vi "Peer to Peer - Basic.vi"() -> ()   [LabVIEW 2023]
uses:
  <vilib>/userDefined/High Color/nirio_resource_hc.ctl
  <vilib>/userDefined/niP2PState.ctl
  <vilib>/FPGAPlugInAG/PXIe-7965R/niLvFpga_Open_PXIe-7965R.vi
  <vilib>/FPGAPlugInAG/PXIe-7965R/niLvFpga_P2PGetEndpoint_PXIe-7965R.vi
  <vilib>/Utility/error.llb/Error Cluster From Error Code.vi
  <vilib>/rvi/errors/niLvFpgaAdjustHostInterfaceError.vi
  <vilib>/FPGAPlugInAG/PXIe-7965R/niLvFpga_Close_PXIe-7965R.vi
  <vilib>/rvi/interface/nirviOpenFPGA/nirviOpenFPGA.xnode
  FPGA Bitfiles/PeerToPeerW_PXIe-7965R.lvbitx
  FPGA Bitfiles/PeerToPeerR_PXIe-7965R.lvbitx
  <vilib>/rvi/interface/nirviMethod/nirviMethod.xnode
  <vilib>/rvi/interface/nirviReadWriteControl/nirviReadWriteControl.xnode
  <vilib>/rvi/interface/nirviCloseFPGA/nirviCloseFPGA.xnode
  <resource>/objmgr/PeerToPeerStream.rc
  <vilib>/rvi/errors/niLvFpgaMergeErrorWithErrorCode.vi
  NiFpgaLv.dll
panel:
  out "Stream State":T1
  in  "Reader":T2="RIO1"
  in  "Writer":T2="RIO0"
  out "Transfer Rate (MB/s)":dbl format="%.3f"
  out "Data Valid?":bool
  out "DataRead":u64
  out "Data Expected":u64
  in  "stop":bool
  in  "Enable":bool
  in  "Flush And Disable":bool
  # "This example shows how to setup and configure a peer to \npeer stream between two PXIe FlexRIO boards. There is a \npeer to peer stream created between the writer and reader \ndevice and once it is enabled, the writer will write a counter \nvalue to the reader. The reader will validate the received\ndata against it's own counter to ensure they match. In \naddition, this example measures throughput of the stream."
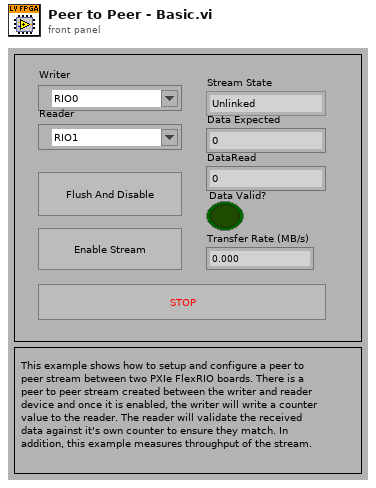
[diagram p1: front panel]
types:
  T1 = typedef "niP2PState.ctl" = enum32{"Unlinked", "Disabled", "Enabled", "Flushing"}
  T2 = typedef "nirio_resource_hc.ctl" = tag
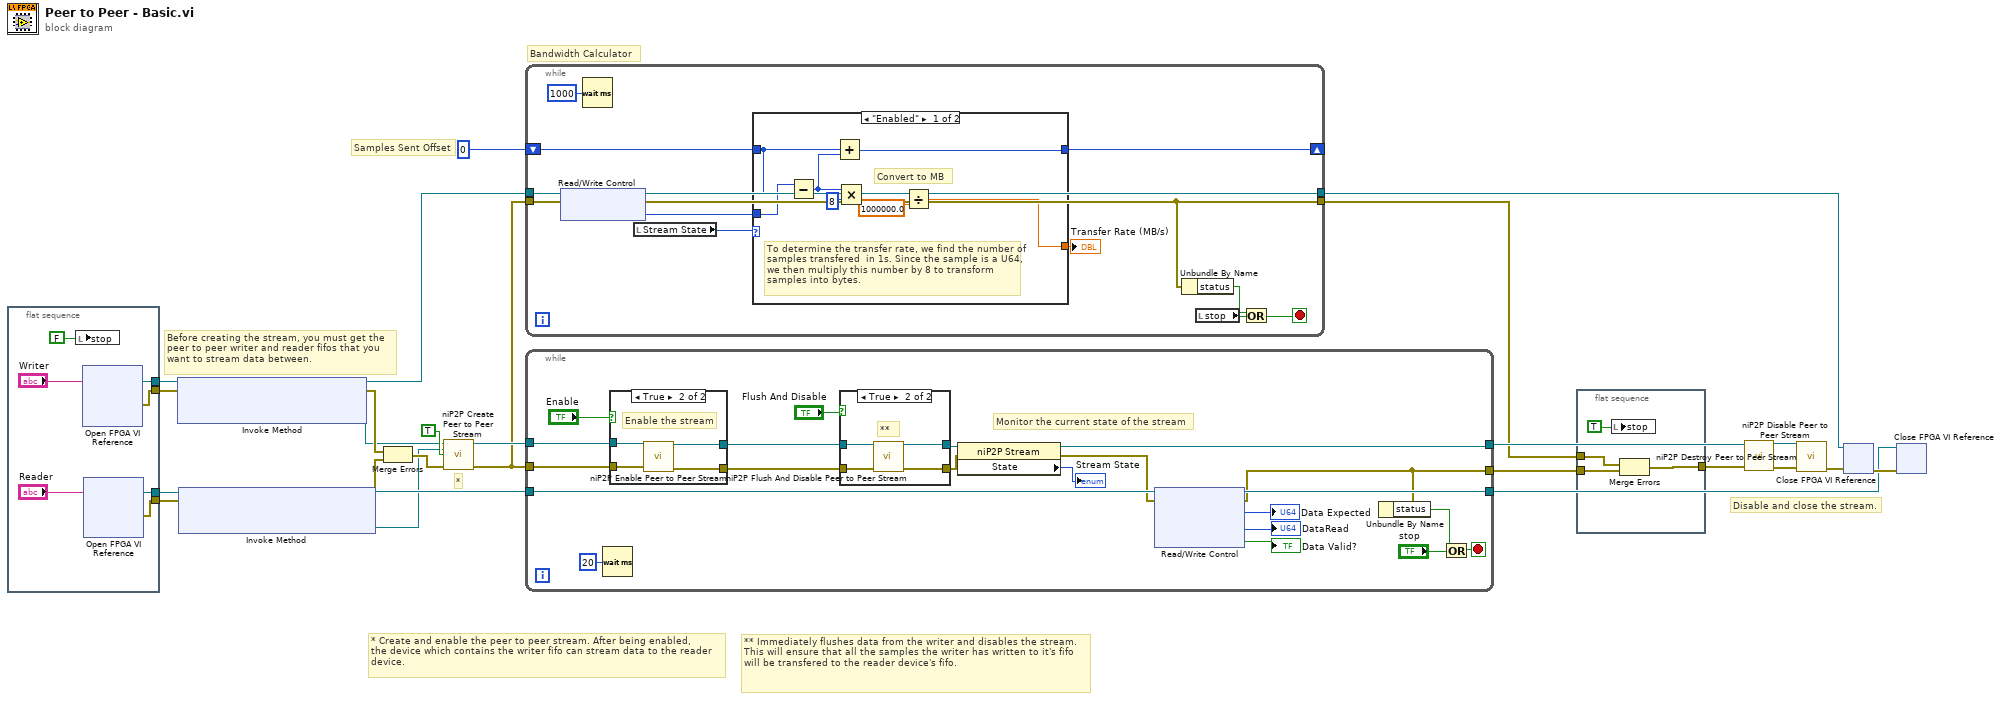
[diagram p0: block diagram]
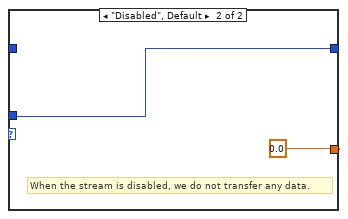
[diagram p2: hidden frame]
diagram:
  # "Bandwidth Calculator"
  # "Samples Sent Offset"
  # "** Immediately flushes data from the writer and disables the stream. \nThis will ensure that all the samples the writer has written to it's fifo \nwill be transfered to the reader device's fifo."
  # "Disable and close the stream."
  # "*"
  # "* Create and enable the peer to peer stream. After being enabled, \nthe device which contains the writer fifo can stream data to the reader\ndevice."
  # "Before creating the stream, you must get the \npeer to peer writer and reader fifos that you \nwant to stream data between."
  n1 = flat-sequence {
    tunnel: [w32] -> w6
    tunnel: [w31] -> w5
    tunnel: [w30] -> w25
    tunnel: [w29] -> w24
    frame #0 {
      n2 = local write "stop"(FALSE ("stop")) -> ()
      n3 = xnode "Open FPGA VI Reference"("resource name"="Writer") -> ("FPGA VI Reference Out"=w32:refnum<k20>, "error out"=w31:errorcluster)  [unwired: 1 in]
      n4 = xnode "Open FPGA VI Reference"("resource name"="Reader") -> ("FPGA VI Reference Out"=w30:refnum<k20>, "error out"=w29:errorcluster)  [unwired: 1 in]
    }
  }
  n5 = xnode "Invoke Method"("FPGA VI Reference In"=w6, "error in"=w5) -> ("FPGA VI Reference Out"=w4:refnum<k20>, "error out"=w3:errorcluster, "Writer"=w2:refnum<k20>)
  n6 = xnode "Invoke Method"("FPGA VI Reference In"=w25, "error in"=w24) -> ("FPGA VI Reference Out"=w23:refnum<k20>, "error out"=w22:errorcluster, "Reader"=w1:refnum<k20>)
  n7 = Merge Errors(w3, w22) -> (w21:errorcluster)
  n8 = call <vilib>:"niP2P Create Peer to Peer Stream.vi"("writer"=w2, "reader"=w1, "enable stream (T)"=TRUE, "error in (no error)"=w21) -> ("stream session"=w13:refnum<k20>, "error out"=w12:errorcluster)  [unwired: 10 in]
  n9 = while {
    tunnel: w4 -> [w39]
    tunnel: w12 -> [w38]
    shift-right: [w40] -> _
    shift-left: u64 0 -> [w41]
    tunnel: [w35] -> w8
    tunnel: [w37] -> w7
    stop <- w43 stop-if-true
    n10 = xnode "Read/Write Control"("FPGA VI Reference In"=w39, "error in"=w38) -> ("FPGA VI Reference Out"=w37:refnum<k20>, "error out"=w35:errorcluster, "Samples Sent"=w33:u64)
    n11 = Wait (ms)(milliseconds to wait=u32 1000) -> ()  [unwired: 1 out]
    n12 = local read "Stream State"() -> (w42:T1)
    n13 = case shown="\"Enabled\"" w42 {
      tunnel: [w49 0.0] -> w45
      tunnel: w41 -> [w48 _]
      tunnel: [w46 w54] -> w40
      tunnel: w33 -> [w53 w54]
      frame "Enabled" {
        # "Convert to MB"
        # "To determine the transfer rate, we find the number of samples transfered  in 1s. Since the sample is a U64, we then multiply this number by 8 to transform samples into bytes."
        n14 = Subtract(x=w53, y=w48) -> (x-y=w47:u64)
        n15 = Add(x=w48, y=w47) -> (x+y=w46:u64)
        n16 = Multiply(x=w47, y=u64 8) -> (x*y=w52:u64)
        n17 = Divide(x=w52, y=1000000.0) -> (x/y=w49:dbl)
      }
      frame "Disabled", Default {
        # "When the stream is disabled, we do not transfer any data."
      }
    }
    "Transfer Rate (MB/s)" <- w45
    n18 = Unbundle By Name(w35) -> ("status"=w34:bool)
    n19 = local read "stop"() -> (w44:bool)
    n20 = Or(x=w34, y=w44) -> (x .or. y?=w43:bool)
  }
  n21 = while {
    tunnel: w13 -> [w74]
    tunnel: w12 -> [w73]
    tunnel: [w62] -> w11
    tunnel: [w58] -> w16
    tunnel: w23 -> [w67]
    tunnel: [w63] -> w19
    stop <- w68 stop-if-true
    # "Monitor the current state of the stream"
    n22 = Wait (ms)(milliseconds to wait=u32 20) -> ()  [unwired: 1 out]
    n23 = case shown="True" "Enable" {
      tunnel: w74 -> [w84 w88]
      tunnel: w73 -> [w83 w87]
      tunnel: [w84 w86] -> w72
      tunnel: [w83 w85] -> w71
      frame False {
      }
      frame True {
        # "Enable the stream"
        n24 = call <vilib>:"niP2P Enable Peer to Peer Stream.vi"("stream session"=w88, "error in (no error)"=w87) -> ("stream session out"=w86:refnum<k20>, "error out"=w85:errorcluster)  [unwired: 12 in]
      }
    }
    n25 = case shown="True" "Flush And Disable" {
      tunnel: w72 -> [w78 w82]
      tunnel: w71 -> [w77 w81]
      tunnel: [w78 w80] -> w60
      tunnel: [w77 w79] -> w59
      frame False {
      }
      frame True {
        # "**"
        n26 = call <vilib>:"niP2P Flush And Disable Peer to Peer Stream.vi"("stream session"=w82, "error in (no error)"=w81) -> ("stream session out"=w80:refnum<k20>, "error out"=w79:errorcluster)  [unwired: 11 in, 1 out]
      }
    }
    n27 = property class="niP2P Stream"(reference=w60, error in=w59) -> (reference out=w58:refnum<k20>, error out=w57:errorcluster, "State"=→"Stream State":T1)
    n28 = xnode "Read/Write Control"("FPGA VI Reference In"=w67, "error in"=w57) -> ("FPGA VI Reference Out"=w63:refnum<k20>, "error out"=w62:errorcluster, "Data Expected"=→"Data Expected":u64, "Data Read"=→"DataRead":u64, "Data Valid?"=→"Data Valid?":bool)
    n29 = Unbundle By Name(w62) -> ("status"=w69:bool)
    n30 = Or(x=w69, y="stop") -> (x .or. y?=w68:bool)
  }
  n31 = flat-sequence {
    tunnel: w11 -> [w92]
    tunnel: [w91] -> w10
    tunnel: w8 -> [w89]
    frame #0 {
      n32 = local write "stop"(TRUE ("stop")) -> ()
      n33 = Merge Errors(w89, w92) -> (w91:errorcluster)
    }
  }
  n34 = call <vilib>:"niP2P Disable Peer to Peer Stream.vi"("stream session"=w16, "error in (no error)"=w10) -> ("stream session out"=w15:refnum<k20>, "error out"=w14:errorcluster)  [unwired: 12 in]
  n35 = call <vilib>:"niP2P Destroy Peer to Peer Stream.vi"("stream session"=w15, "error in (no error)"=w14) -> ("error out"=w18:errorcluster)  [unwired: 13 in]
  n36 = xnode "Close FPGA VI Reference"("FPGA VI Reference In"=w7, "error in"=w18) -> ("error out"=w20:errorcluster)
  n37 = xnode "Close FPGA VI Reference"("FPGA VI Reference In"=w19, "error in"=w20) -> ()  [unwired: 1 out]
